vi "Conpane Wrapper Demo.vi"() -> ()   [LabVIEW 2018]
uses:
  Subvis/Term Types.ctl
  Subvis/Term Type.ctl
  Subvis/conpane_test.vi
  ConPane Wrapper.xnode
panel:
  out "Numeric 2":dbl
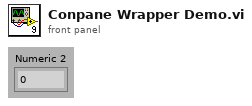
[diagram p1: front panel]
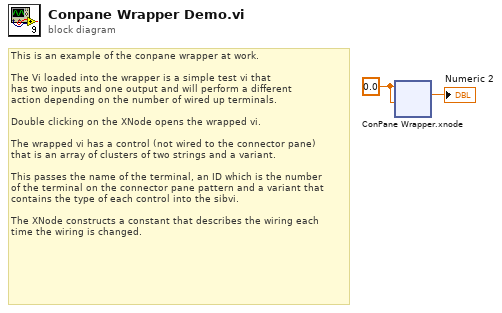
[diagram p0: block diagram]
diagram:
  w1 = 0.0 ("Numeric")
  # "This is an example of the conpane wrapper at work.\n\nThe Vi loaded into the wrapper is a simple test vi that\nhas two inputs and one output and will perform a different\naction depending on the number of wired up terminals.\n\nDouble clicking on the XNode opens the wrapped vi.\n\nThe wrapped vi has a control (not wired to the connector pane)\nthat is an array of clusters of two strings and a variant.\n\nThis passes the name of the terminal, an ID which is the number\nof the terminal on the connector pane pattern and a variant that\ncontains the type of each control into the sibvi.\n\nThe XNode constructs a constant that describes the wiring each\ntime the wiring is changed."
  n1 = xnode "ConPane Wrapper.xnode"("Numeric 3"=w1, "Numeric"=w1) -> ("Numeric 2"=→"Numeric 2":dbl)
